vi "Create Channel Array.vi"(8 "error in":errorcluster, 9 "expected channel count":i32, 10 "channel settings":T1[](array[typedef]), 11 "counter driven output mode in":refnum<class "Counter Driven Output Mode.lvclass">) -> (0 "error out":errorcluster, 2 "channels":refnum<class "Counter Driven Output Channel.lvclass">[](array[class]), 3 "counter driven output mode out":refnum<class "Counter Driven Output Mode.lvclass">)   [LabVIEW 2017, in "Scan Engine Scripting.lvlib" / "Counter Driven Output Mode.lvclass"]
uses:
  Counter Driven Output Mode.lvclass
  Controls/counter driven output channel settings.ctl
  Channel Classes/Counter Driven Output Channel/Counter Driven State.ctl
  Channel Classes/Counter Driven Output Channel/Counter Driven Output Channel.lvclass
  Scan Engine Scripting.lvlib
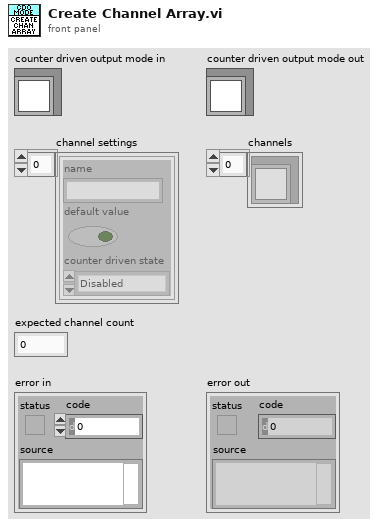
[diagram p1: front panel]
types:
  T1 = typedef "Scan Engine Scripting.lvlib/counter driven output channel settings.ctl" = cluster{"name":string, "default value":bool, "counter driven state":T2}
  T2 = typedef "Scan Engine Scripting.lvlib/Counter Driven Output Channel.lvclass/Counter Driven State.ctl" = enum16{"Disabled", "Enabled"}
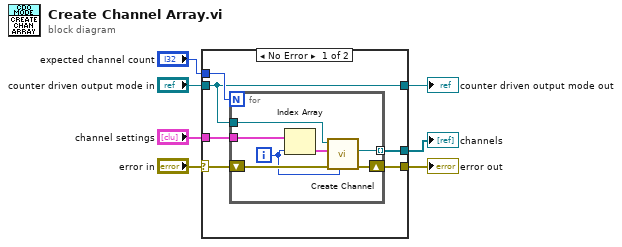
[diagram p0: block diagram]
diagram:
  n1 = case shown="No Error" "error in" {
    selector: "error in" -> [w11 w22]
    tunnel: [w10 w22] -> w6
    tunnel: [w12 w21] -> w4
    tunnel: "counter driven output mode in" -> [w12 w21]
    tunnel: "expected channel count" -> [w13 _]
    tunnel: "channel settings" -> [w9 _]
    tunnel: [w8 _] -> w1
    frame No Error {
      n2 = for {
        N: w13 -> [_]
        tunnel: w12 -> [w20]
        tunnel: w9 -> [w17]
        shift-right: [w18] -> w10
        shift-left: w11 -> [w19]
        tunnel: [w14] -> w8 mode=indexing
        i -> [w15]
        n3 = Index Array(array=w17, index=w15) -> (element=w16:T1)
        n4 = call "Create Channel.vi"("index"=w15, "error in"=w19, "channel settings"=w16, "counter driven output mode in"=w20) -> ("error out"=w18:errorcluster, "counter driven output channel out"=w14:refnum<class "Counter Driven Output Channel.lvclass">)  [unwired: 5 in, 1 out]
      }
    }
    frame Error {
    }
  }
  "error out" <- w6
  "counter driven output mode out" <- w4
  "channels" <- w1
